vi "can_initialize.vi"(8 "error in (no error)":errorcluster, 11 "Instrument in":refnum<class "Instrument.lvclass">) -> (0 "error out":errorcluster, 3 "Instrument out":refnum<class "Instrument.lvclass">)   [LabVIEW 2019, in "Instrument.lvclass"]
uses:
  Instrument.lvclass
  Instrument.lvclass/Instrument.ctl
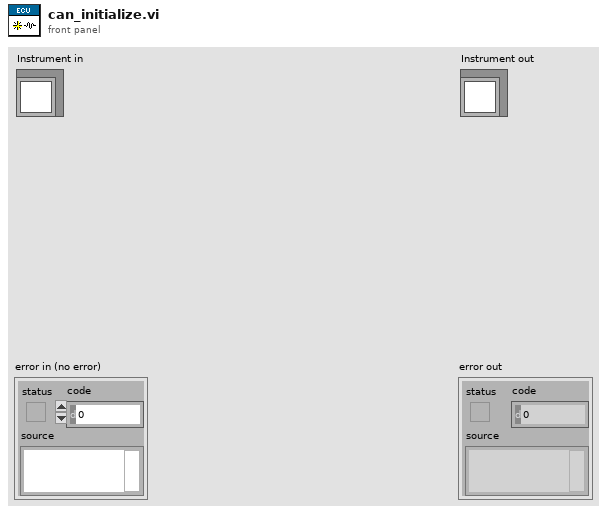
[diagram p1: front panel]
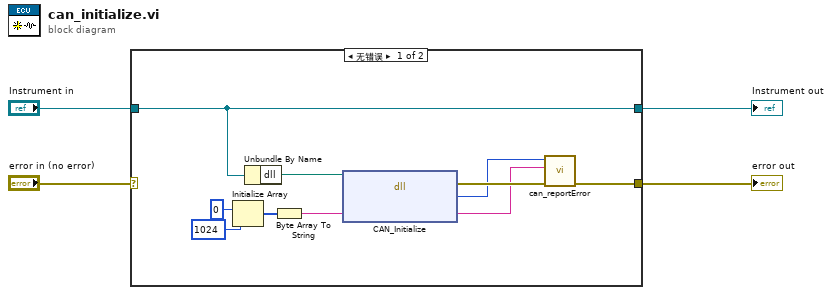
[diagram p0: block diagram]
diagram:
  n1 = case shown="无错误" "error in (no error)" {
    selector: "error in (no error)" -> [_ w16]
    tunnel: [w9 w16] -> w3
    tunnel: [w14 w15] -> w1
    tunnel: "Instrument in" -> [w14 w15]
    frame No Error {
      n2 = Initialize Array(u8 0 ("element"), 1024 ("dimension size")) -> (w6:u8[])
      n3 = Unbundle By Name(w14) -> ("dll"=w13:path)
      n4 = Byte Array To String(unsigned byte array=w6) -> (string=w5:string)
      n5 = dll-call lib="C:/Dev/22KW-Dyno/software/data/DynoAPI.dll" fn="CAN_Initialize"(path in=w13, "ErrorMsg"=w5) -> (error out=w12:errorcluster, "return type"=w11:i32, "ErrorMsg"=w10:string)  [unwired: 2 in, 1 out]
      n6 = call "can_reportError.vi"("error in (no error)"=w12, "errorMsg"=w10, "return type"=w11) -> ("error out"=w9:errorcluster)  [unwired: 8 in]
    }
    frame Error {
    }
  }
  "error out" <- w3
  "Instrument out" <- w1
